vi "Delete Tree.vi"(8 "error in (no error)":errorcluster, 11 "UA Server in":refnum<class "UA Server.lvclass">) -> (0 "error out":errorcluster)   [LabVIEW 2017, in "Browser Core.lvlib" / "UA Server.lvclass"]
doc: "Use this as the destructor for the tree object"
uses:
  UA Server.lvclass
  UA Server.lvclass/UA Server.ctl
  <vilib>/OPCUA/NI OPC UA Client.lvlib
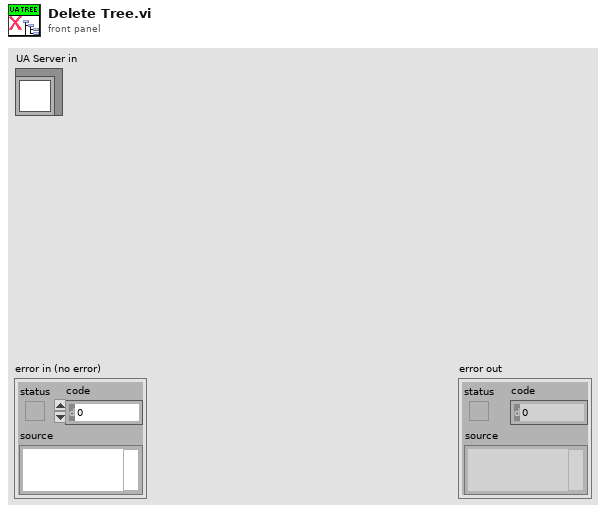
[diagram p1: front panel]
types:
  T1 = typedef "OPC UA Client Refnum.ctl" = refnum<k21>
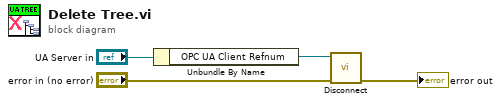
[diagram p0: block diagram]
diagram:
  n1 = Unbundle By Name("UA Server in") -> ("OPC UA Client Refnum"=w3:T1)
  n2 = call <vilib>:"Disconnect.vi"("error in (no error)"="error in (no error)", "OPC UA client refnum in"=w3) -> ("error out"=→"error out":errorcluster)  [unwired: 9 in]
